vi "getUiControlsRefnums.vi"(8 "error in (no error)":errorcluster, 10 "Control Indexes":string[](array[string]), 11 "uiControlsMgr in":refnum<class "uiControlsMgr.lvclass">) -> (0 "error out":errorcluster, 2 "Control Refnums":refnum<vi>[](array[refnum]), 3 "uiControlsMgr out":refnum<class "uiControlsMgr.lvclass">)   [LabVIEW 2020, in "UI Controls Manager.lvlib" / "uiControlsMgr.lvclass"]
uses:
  uiControlsMgr.lvclass
  uiControlsMgr.lvclass/uiControlsMgr.ctl
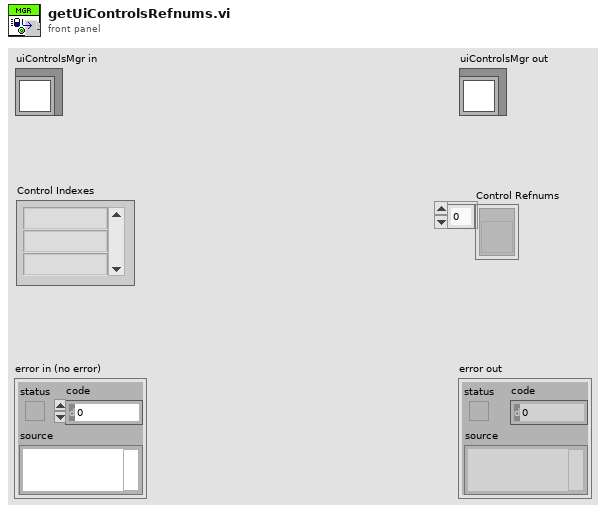
[diagram p1: front panel]
types:
  T1 = map{string, cluster{"Caption":string, "Ctl Refnum":refnum<vi>}}
  T2 = cluster{"Caption":string, "Ctl Refnum":refnum<vi>}
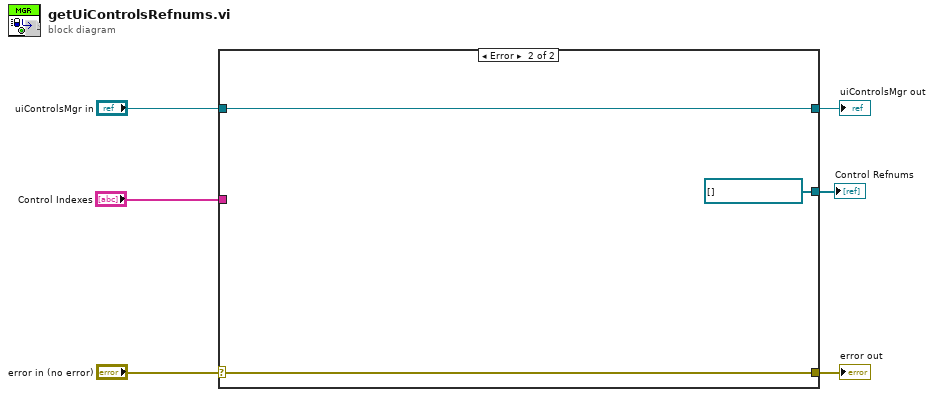
[diagram p0: block diagram]
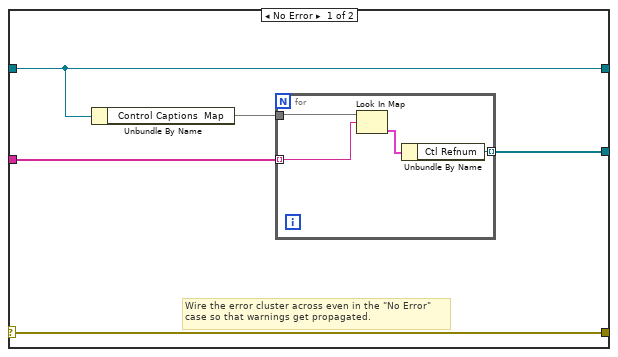
[diagram p2: hidden frame]
diagram:
  n1 = case shown="Error" "error in (no error)" {
    selector: "error in (no error)" -> [w11 w18]
    tunnel: [w11 w18] -> w5
    tunnel: [w10 w17] -> w3
    tunnel: "uiControlsMgr in" -> [w10 w17]
    tunnel: "Control Indexes" -> [w9 _]
    tunnel: [w7 refnum<vi>[] []] -> w1
    frame No Error {
      # "Wire the error cluster across even in the \"No Error\"\ncase so that warnings get propagated."
      n2 = Unbundle By Name(w10) -> ("Control Captions  Map"=w8:T1)
      n3 = for {
        tunnel: w9 -> [w14] mode=indexing
        tunnel: w8 -> [w15]
        tunnel: [w12] -> w7 mode=indexing
        n4 = Look In Map(map=w15, key=w14) -> (value=w13:T2)  [unwired: 1 in, 1 out]
        n5 = Unbundle By Name(w13) -> ("Ctl Refnum"=w12:refnum<vi>)
      }
    }
    frame Error {
    }
  }
  "error out" <- w5
  "uiControlsMgr out" <- w3
  "Control Refnums" <- w1
